vi "NI VeriStand - Get Next Unique Label.vi"(7 "format string":string=" %d", 8 "error in (no error)":errorcluster, 9 "Start Value (1)":i32=1, 10 "Label":string, 11 "Parent Ref in":T1=18446744073709551615 format="%.0x") -> (0 "error out":errorcluster, 2 "Label out":string, 3 "Parent Ref dup":T1=18446744073709551615 format="%.0x", 4 "Next value":i32)   [LabVIEW 2020, in "Custom Device Utility Library.lvlib"]
doc: "Searches under the <B>Parent Ref</B> you specify for a base <B>Label</B> you specify and returns the next valid, or unused, full label that uses that base. This VI assumes that a valid full label is the base label with an incremented number appended to it."
uses:
  <vilib>/NI VeriStand/Custom Device Tools/Custom Device Utility Library/Custom Device Utility Library.lvlib
  <vilib>/NI VeriStand/Custom Device API/Custom Device Item Ref.ctl
  <vilib>/NI VeriStand/Custom Device API/Custom Device API.lvlib
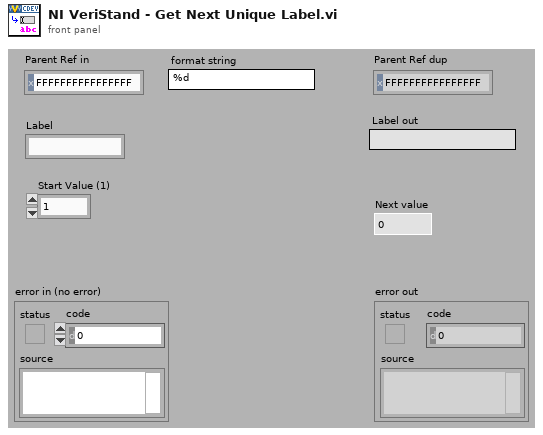
[diagram p1: front panel]
types:
  T1 = typedef "Custom Device API.lvlib/Custom Device Item Ref.ctl" = u64
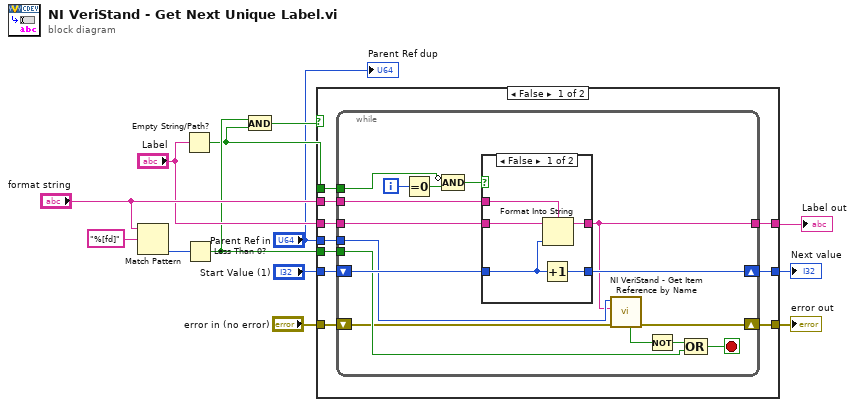
[diagram p0: block diagram]
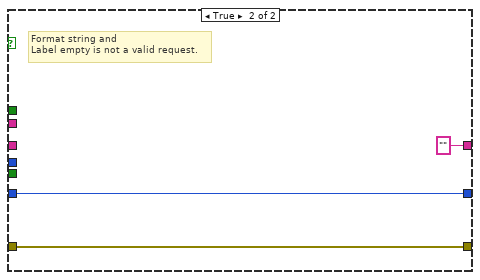
[diagram p3: hidden frame]
diagram:
  n1 = Match Pattern(string="format string", regular expression="%[fd]") -> (offset past match=w10:i32)  [unwired: 1 in, 3 out]
  n2 = Empty String/Path?(string/path="Label") -> (empty?=w6:bool)
  n3 = Less Than 0?(x=w10) -> (x < 0?=w7:bool)
  n4 = And(x=w7, y=w6) -> (x .and. y?=w5:bool)
  n5 = case shown="False" w5 {
    tunnel: "Parent Ref in" -> [w23 _]
    tunnel: [w22 "" ("Label")] -> w13
    tunnel: "Start Value (1)" -> [w21 w48]
    tunnel: "format string" -> [w20 _]
    tunnel: w7 -> [w19 _]
    tunnel: "Label" -> [w18 _]
    tunnel: w6 -> [w17 _]
    tunnel: [w16 w48] -> w8
    tunnel: "error in (no error)" -> [w15 w47]
    tunnel: [w14 w47] -> w2
    frame False {
      n6 = while {
        shift-right: [w28] -> w16
        shift-left: w21 -> [w39]
        tunnel: w18 -> [w38]
        tunnel: w23 -> [w27]
        tunnel: [w26] -> w22
        tunnel: w20 -> [w37]
        tunnel: w19 -> [w31]
        tunnel: w17 -> [w29]
        shift-right: [w24] -> w14
        shift-left: w15 -> [w25]
        i -> [w35]
        stop <- w32 stop-if-true
        n7 = Equal To 0?(x=w35) -> (x = 0?=w36:bool)
        n8 = Compound Arithmetic op=AND(invert w29, w36) -> (w30:bool)
        n9 = case shown="False" w30 {
          tunnel: w39 -> [w41 w45]
          tunnel: [w44 w46] -> w26
          tunnel: w38 -> [w43 w46]
          tunnel: w37 -> [w42 _]
          tunnel: [w40 w45] -> w28
          frame False {
            n10 = Increment(x=w41) -> (x+1=w40:i32)
            n11 = Format Into String(format string=w42, initial string=w43, w41) -> (resulting string=w44:string)  [unwired: 1 in, 1 out]
          }
          frame True {
          }
        }
        n12 = call <vilib>:"NI VeriStand - Get Item Reference by Name.vi"("error in (no error)"=w25, "Item Name"=w26, "Parent Ref in"=w27) -> ("error out"=w24:errorcluster, "Found"=w34:bool)  [unwired: 5 in, 2 out]
        n13 = Not(x=w34) -> (.not. x?=w33:bool)
        n14 = Compound Arithmetic op=OR(w33, w31) -> (w32:bool)
      }
    }
    frame True {
      # "Format string and\nLabel empty is not a valid request."
    }
  }
  "Label out" <- w13
  "error out" <- w2
  "Next value" <- w8
  "Parent Ref dup" <- "Parent Ref in"
